vi "Add Contestant.vi"(8 "error in (no error)":errorcluster, 9 "Position":i32, 10 "Name":string, 11 "Controller in":refnum<class "Controller.lvclass">) -> (0 "error out":errorcluster, 3 "Controller out":refnum<class "Controller.lvclass">)   [LabVIEW 2024, in "Controller.lvlib" / "Controller.lvclass"]
uses:
  Controller.lvclass
  Applications/National Instruments/LabVIEW 2024 64-bit/vi.lib/ActorFramework/Actor/Actor.lvclass
  Controller.lvclass/Controller.ctl
  Contestant/Contestant/Contestant.lvclass
  <vilib>/ActorFramework/Actor/Actor.lvclass
  Users/elijahkerry/challenge-of-champions/Contestant/Contestant/Contestant.lvclass
  Users/elijahkerry/challenge-of-champions/Controller/Controller/Controller.lvclass
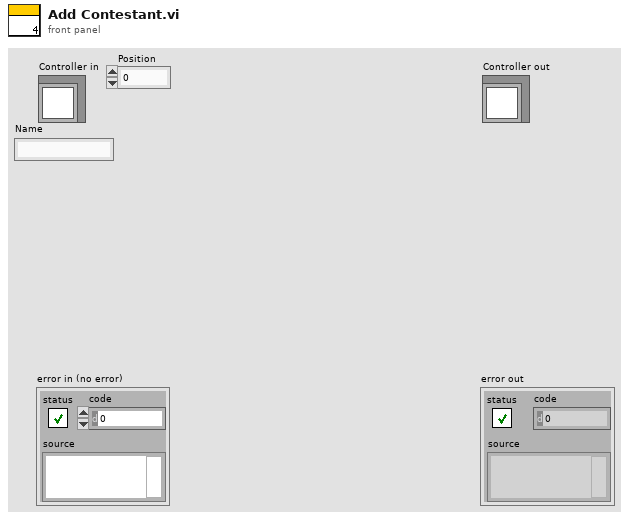
[diagram p1: front panel]
types:
  T1 = map{i32, refnum<class "Message Enqueuer.lvclass">}
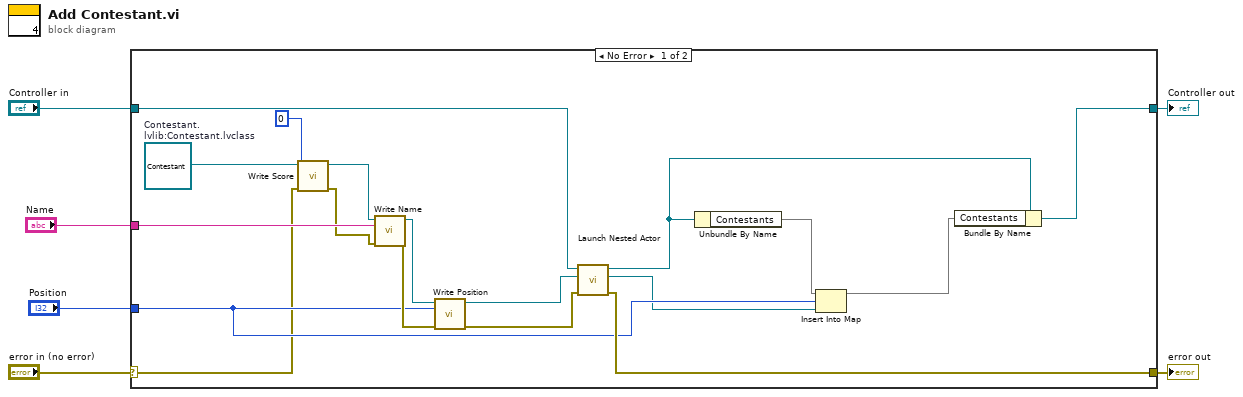
[diagram p0: block diagram]
diagram:
  n1 = case shown="No Error" "error in (no error)" {
    selector: "error in (no error)" -> [w8 w26]
    tunnel: [w23 w26] -> w5
    tunnel: [w12 w25] -> w3
    tunnel: "Controller in" -> [w24 w25]
    tunnel: "Name" -> [w18 _]
    tunnel: "Position" -> [w17 _]
    frame No Error {
      w11 = refnum<class "Contestant.lvclass"> refnum  # Contestant.lvlib:Contestant.lvclass
      n2 = call "Write Score.vi"("error in (no error)"=w8, "Score"=0, "Contestant in"=w11) -> ("error out"=w7:errorcluster, "Contestant out"=w10:refnum<class "Contestant.lvclass">)  [unwired: 7 in]
      n3 = call-dynamic "Write Name.vi"("error in (no error)"=w7, "Name"=w18, "Contestant in"=w10) -> ("error out"=w20:errorcluster, "Contestant out"=w22:refnum<class "Contestant.lvclass">)  [unwired: 7 in]
      n4 = call-dynamic "Write Position.vi"("error in (no error)"=w20, "Position"=w17, "Contestant in"=w22) -> ("error out"=w19:errorcluster, "Contestant out"=w21:refnum<class "Contestant.lvclass">)  [unwired: 7 in]
      n5 = call <vilib>:"Launch Nested Actor.vi"("error in (no error)"=w19, "Nested Actor"=w21, "Caller Actor in"=w24) -> ("error out"=w23:errorcluster, "Nested Actor's Enqueuer"=w16:refnum<class "Message Enqueuer.lvclass">, "Caller Actor out"=w14:refnum<class "Controller.lvclass">)  [unwired: 6 in]
      n6 = Unbundle By Name(w14) -> ("Contestants"=w15:T1)
      n7 = Insert Into Map(map in=w15, key=w17, value=w16) -> (map out=w13:T1)  [unwired: 2 out]
      n8 = Bundle By Name(cluster=w14, "Contestants"=w13) -> (w12:refnum<class "Controller.lvclass">)
    }
    frame Error {
    }
  }
  "error out" <- w5
  "Controller out" <- w3
